vi "Update All DUT Statuses.vi"(8 "error in (no error)":errorcluster, 9 "BG Color":u32(colorbox), 10 "Message ('')":string, 11 "Application in":refnum<class "Application.lvclass">) -> (0 "error out":errorcluster, 3 "Application out":refnum<class "Application.lvclass">)   [LabVIEW 2017, in "Application.lvlib" / "Application.lvclass"]
doc: "Updates all positions status messages with the \"Message\" and \"BG Color\" regardless of state."
uses:
  Application.lvclass
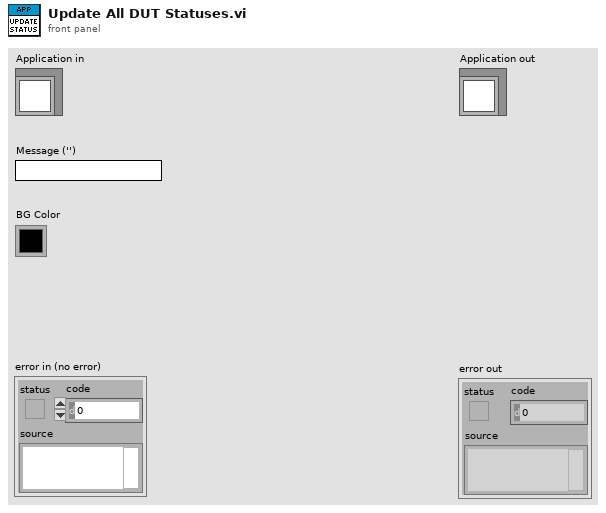
[diagram p1: front panel]
types:
  T1 = typedef "Application.lvlib/App Properties.lvclass/Class Properties -- Cluster.ctl" = cluster{"UUT Info":T2[], "Test Information":refnum<vi>, "Gold Board":refnum<class "Golden Board.lvclass">, "Test Recipe":refnum<class "Test Recipe.lvclass">, "Instruments":refnum<class "Instrument.lvclass">[], "Mode":T3, "Test Results":T4[], "Station Config":refnum<class "Station Config.lvclass">, "Variable Engine":refnum<class "Variable Engine.lvclass">}
  T2 = typedef "Application.lvlib/App Properties.lvclass/UUT Reference -- Cluster.ctl" = cluster{"Serial Number Reference":refnum<vi>, "Status Message Reference":refnum<vi>}
  T3 = typedef "Application.lvlib/Application.lvclass/Op Mode -- Enum.ctl" = u16
  T4 = typedef "Application.lvlib/App Properties.lvclass/Test Result -- Cluster.ctl" = cluster{"Position":i32, "Pass":bool, "Fail Codes":string}
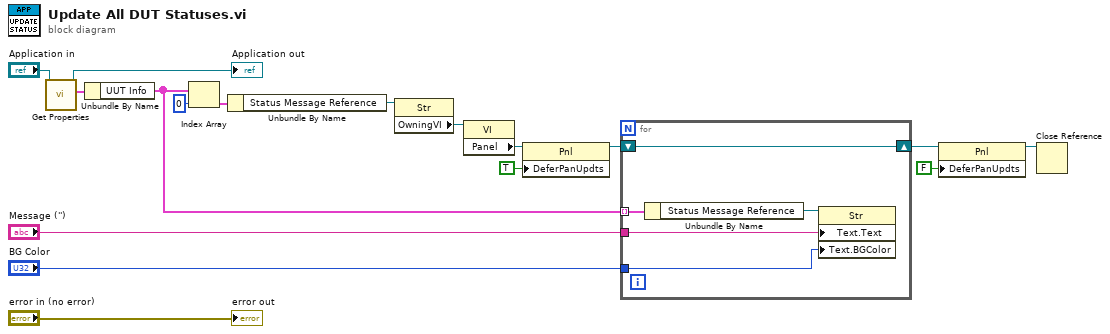
[diagram p0: block diagram]
diagram:
  n1 = call "Get Properties.vi"("Acrobat Template in"="Application in") -> ("Class Properties"=w12:T1, "Acrobat Template out"=→"Application out":refnum<class "Application.lvclass">)  [unwired: 8 in, 1 out]
  n2 = Unbundle By Name(w12) -> ("UUT Info"=w5:T2[])
  n3 = Index Array(array=w5, index=0) -> (element=w6:T2)
  n4 = Unbundle By Name(w6) -> ("Status Message Reference"=w10:refnum<vi>)
  n5 = property class="Str"(reference=w10) -> ("OwningVI"=w9:refnum<vi>)  [unwired: 1 in, 2 out]
  n6 = property class="VI"(reference=w9) -> ("Panel"=w8:refnum<vi>)  [unwired: 1 in, 2 out]
  n7 = property class="Pnl"(reference=w8, "DeferPanUpdts"=TRUE ("Defer Panel Updates")) -> (reference out=w4:refnum<vi>)  [unwired: 1 in, 1 out]
  n8 = for {
    tunnel: "Message ('')" -> [w22]
    tunnel: "BG Color" -> [w21]
    tunnel: w5 -> [w19] mode=indexing
    shift-right: [w18] -> w2
    shift-left: w4 -> [w18]
    n9 = Unbundle By Name(w19) -> ("Status Message Reference"=w20:refnum<vi>)
    n10 = property class="Str"(reference=w20, "Text.Text"=w22, "Text.BGColor"=w21) -> ()  [unwired: 1 in, 2 out]
  }
  n11 = property class="Pnl"(reference=w2, "DeferPanUpdts"=FALSE ("Defer Panel Updates")) -> (reference out=w1:refnum<vi>)  [unwired: 1 in, 1 out]
  n12 = Close Reference(reference=w1) -> ()  [unwired: 1 in, 1 out]
  "error out" <- "error in (no error)"
